vi "Main Basler.vi"() -> ()   [LabVIEW 2021]
doc: "VI that makes simple snapshot with <b>Basler</b> camera. Inventory ID: 50065895s"
uses:
  <vilib>/vision/driver/NI_Vision_Acquisition_Software.lvlib
panel:
  out "Image":T1(plugin-control)
  in  "Camera Name":refnum<k21> caption="IMAQdx Session"
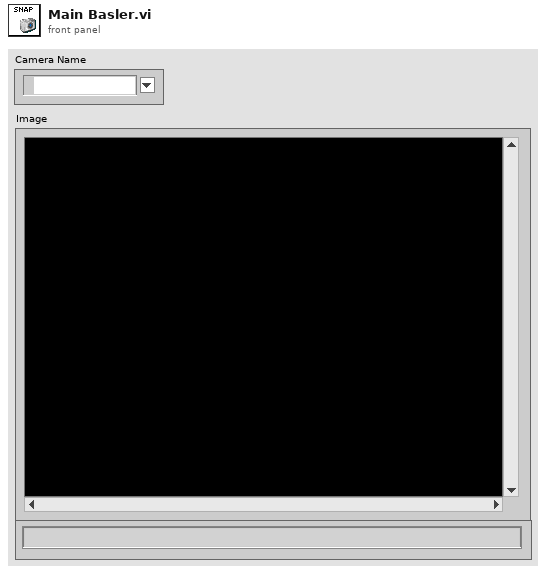
[diagram p1: front panel]
types:
  T1 = typedef "IMAQ Image.ctl" = refnum<image>
  T2 = typedef "Image Type" = u32
  T3 = typedef "IMAQdx.ctl" = refnum<k21>
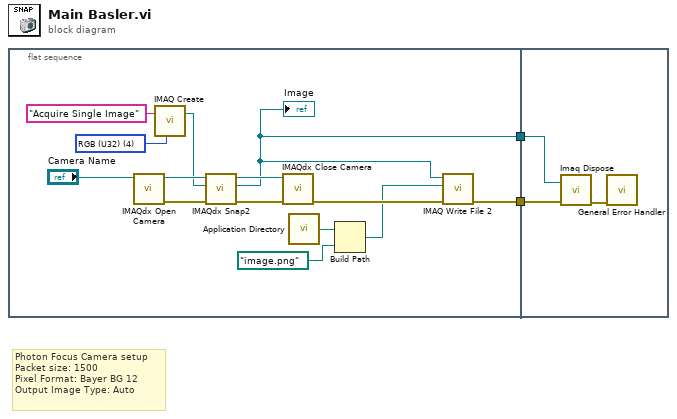
[diagram p0: block diagram]
diagram:
  # "Photon Focus Camera setup\nPacket size: 1500\nPixel Format: Bayer BG 12\nOutput Image Type: Auto"
  n1 = flat-sequence {
    tunnel: [w6] -> w2
    tunnel: [w8] -> w1
    tunnel: w2 -> [w19]
    tunnel: w1 -> [w18]
    frame #0 {
      w9 = T2 4 items=["Grayscale (U8)", "Grayscale (I16)", "Grayscale (SGL)", "Complex (CSG)", "RGB (U32)", "HSL (U32)", "RGB (U64)", "Grayscale (U16)"] ("Image Type")
      n2 = call <vilib>:"IMAQdx Open Camera.vi"("Session In"="Camera Name") -> ("error out"=w12:errorcluster, "Session Out"=w15:T3)  [unwired: 2 in, 7 out]
      n3 = call "IMAQ Create"("Image Name"="Acquire Single Image", "Image Type"=w9) -> ("New Image"=w11:T1)  [unwired: 2 in, 2 out]
      n4 = call <vilib>:"IMAQdx Snap2.vi"("error in"=w12, "Image In"=w11, "Session In"=w15) -> ("error out"=w14:errorcluster, "Image Out"=w8:T1, "Session Out"=w16:T3)  [unwired: 6 in]
      "Image" <- w8
      n5 = call <vilib>:"IMAQdx Close Camera.vi"("error in"=w14, "Session In"=w16) -> ("error out"=w7:errorcluster)  [unwired: 9 out]
      n6 = call <vilib>:"Application Directory.vi"() -> ("Application Directory"=w5:path)
      n7 = Build Path(base path=w5, name or relative path=path "image.png") -> (appended path=w4:path)
      n8 = call-poly "IMAQ Write File 2"("error in (no error)"=w7, "File Path"=w4, "Image"=w8) -> ("error out"=w6:errorcluster)  [unwired: 7 in, 1 out]
    }
    frame #1 {
      n9 = call "Imaq Dispose"("Image"=w18, "error in (no error)"=w19) -> ("error out"=w17:errorcluster)  [unwired: 4 in]
      n10 = call <vilib>:"General Error Handler.vi"("error in (no error)"=w17) -> ()  [unwired: 2 in, 13 out]
    }
  }
